vi "09 Clusters.vi"() -> ()   [LabVIEW 2019]
panel:
  out "Waveform Graph":T1(graph)
  out "Clusters and Plots 2":cluster{i32, "number: 0 to 1":dbl}[](graph)
  out "Clusters and Plots":cluster{i32[], dbl[]}(graph)
  out "fixed 1":T2
  out "fixed 2":T2
  in  "Cluster":T2={"Name"="Al Einstein", "Height (cm)"=170.0, "attended"=FALSE}
  # "Hit the Run arrow and see the code execute"
  # "Right btn click to change \nautomatic arrangement"
  # "Hit Cmd E to see the diagram (code)"
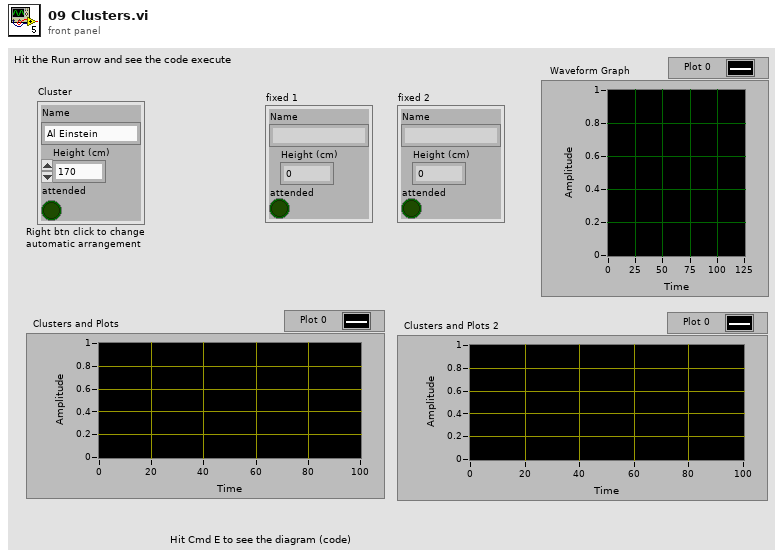
[diagram p1: front panel]
types:
  T1 = cluster{"Height (cm)":dbl, "Height (cm)":dbl, dbl[]}
  T2 = cluster{"Name":string, "Height (cm)":dbl, "attended":bool}
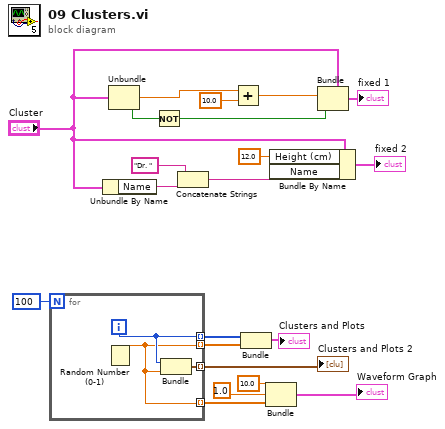
[diagram p0: block diagram]
diagram:
  n1 = for {
    N: 100 -> [_]
    tunnel: [w24] -> w9 mode=indexing
    tunnel: [w22] -> w8 mode=indexing
    tunnel: [w23] -> w5 mode=indexing
    tunnel: [w22] -> w4 mode=indexing
    i -> [w24]
    n2 = Random Number (0-1)() -> (number: 0 to 1=w22:dbl)
    n3 = Bundle(w24, "number: 0 to 1"=w22) -> (w23:cluster{i32, "number: 0 to 1":dbl})  [unwired: 1 in]
  }
  "Clusters and Plots 2" <- w5
  n4 = Unbundle By Name("Cluster") -> ("Name"=w12:string)
  n5 = Unbundle("Cluster") -> ("Height (cm)"=w18:dbl, "attended"=w15:bool)  [unwired: 1 out]
  n6 = Not(x=w15) -> (.not. x?=w14:bool)
  n7 = Concatenate Strings("Dr. " ("string"), w12) -> (w10:string)
  n8 = Add(x=w18, y=10.0) -> (x+y=w16:dbl)
  n9 = Bundle(w9, w8) -> (→"Clusters and Plots":cluster{i32[], dbl[]})  [unwired: 1 in]
  n10 = Bundle("Height (cm)"=10.0, "Height (cm)"=1.0, w4) -> (→"Waveform Graph":T1)  [unwired: 1 in]
  n11 = Bundle By Name(cluster="Cluster", "Height (cm)"=12.0, "Name"=w10) -> (→"fixed 2":T2)
  n12 = Bundle(cluster="Cluster", "Height (cm)"=w16, "attended"=w14) -> (→"fixed 1":T2)  [unwired: 1 in]
